vi "S2C_BldEnterSubScr.vi"(8 "Error In":errorcluster, 11 "Data":string) -> (0 "Error Out":errorcluster)   [LabVIEW 2015]
doc: "Deletes the selected items from the script table."
uses:
  Globals/S2C_Globals.vi
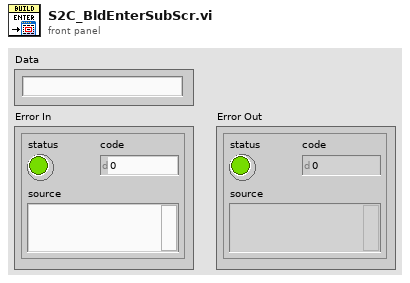
[diagram p1: front panel]
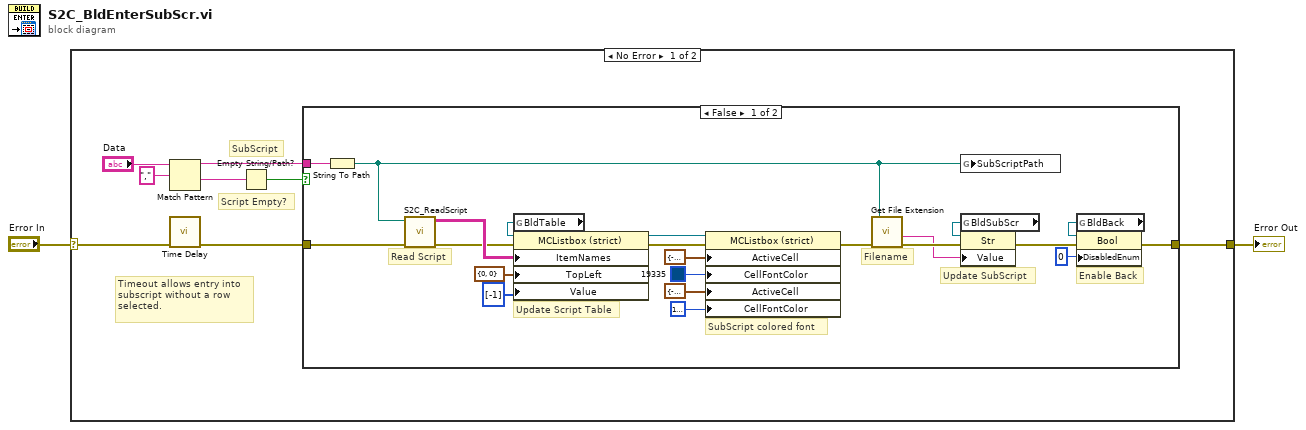
[diagram p0: block diagram]
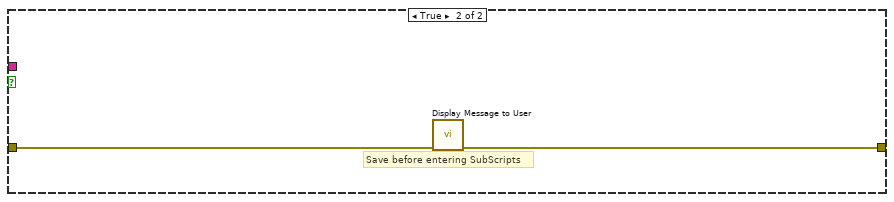
[diagram p2: hidden frame]
diagram:
  n1 = case shown="No Error" "Error In" {
    selector: "Error In" -> [w4 w35]
    tunnel: [w6 w35] -> w1
    frame No Error {
      # "SubScript"
      # "Script Empty?"
      # "Timeout allows entry into\nsubscript without a row\nselected."
      n2 = Match Pattern(string="Data", regular expression=",") -> (before substring=w7:string, after substring=w5:string)  [unwired: 1 in, 2 out]
      n3 = call "Time Delay"("error in (no error)"=w4) -> ("error out"=w3:errorcluster)  [unwired: 10 in]
      n4 = Empty String/Path?(string/path=w5) -> (empty?=w8:bool)
      n5 = case shown="False" w8 {
        tunnel: w3 -> [w14 w34]
        tunnel: w7 -> [w26 _]
        tunnel: [w24 w33] -> w6
        frame False {
          # "Read Script"
          # "SubScript colored font"
          # "Filename"
          # "Update Script Table"
          # "Enable Back"
          # "Update SubScript"
          n6 = String To Path(string=w26) -> (path=w11:path)
          n7 = call "S2C_ReadScript.vi"("Error In"=w14, "FilePath"=w11) -> ("Error Out"=w12:errorcluster, "Data"=w13:string[][])  [unwired: 8 in]
          n8 = global read "S2C_Globals.vi" "BldTable"() -> (w32:refnum<vi>)
          n9 = property class="MCListbox (strict)"(reference=w32, error in=w12, "ItemNames"=w13, "TopLeft"=cluster{"Row":u32, "Column":u32} {"Row"=0, "Column"=0} ("Top Left Visible Cell"), "Value"=i32[] [-1]) -> (reference out=w20:refnum<vi>, error out=w21:errorcluster)
          n10 = property class="MCListbox (strict)"(reference=w20, error in=w21, "ActiveCell"=cluster{"Row":i32, "Column":i32} {"Row"=-2, "Column"=-2} ("Active Cell:Active Cell"), "CellFontColor"=u32 19335, "ActiveCell"=cluster{"Row":i32, "Column":i32} {"Row"=-1, "Column"=-2} ("Active Cell:Active Cell"), "CellFontColor"=u32 16777226) -> (error out=w19:errorcluster)  [unwired: 1 out]
          n11 = call <vilib>:"Get File Extension.vi"("error in (no error)"=w19, "file"=w11) -> ("error out"=w23:errorcluster, "filename without extension"=w22:string)  [unwired: 5 in, 3 out]
          n12 = global write "S2C_Globals.vi" "SubScriptPath"(w11) -> ()
          n13 = global read "S2C_Globals.vi" "BldSubScr"() -> (w29:refnum<vi>)
          n14 = property class="Str"(reference=w29, error in=w23, "Value"=w22) -> (error out=w27:errorcluster)  [unwired: 1 out]
          n15 = global read "S2C_Globals.vi" "BldBack"() -> (w28:refnum<vi>)
          n16 = property class="Bool"(reference=w28, error in=w27, "DisabledEnum"=u8 0) -> (error out=w24:errorcluster)  [unwired: 1 out]
        }
        frame True {
          # "Save before entering SubScripts"
          n17 = call "Display Message to User"("error in (no error)"=w34) -> ("error out"=w33:errorcluster)  [unwired: 9 in, 1 out]
        }
      }
    }
    frame Error {
    }
  }
  "Error Out" <- w1
